vi "fgv_PXI-5110_procon.vi"(7 "cmd":T2, 8 "error in":errorcluster, 11 "data":T1) -> (0 "error out":errorcluster, 3 "queue out":refnum<queue>)   [LabVIEW 2021]
uses:
  ctrl/create-rw-close.ctl
  ctrl/5110_cmd.ctl
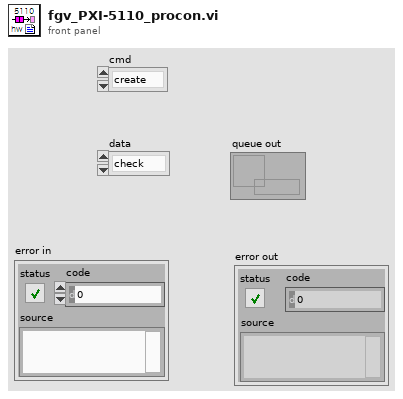
[diagram p1: front panel]
types:
  T1 = typedef "5110_cmd.ctl" = enum16{"check", "run", "stop"}
  T2 = typedef "create-rw-close.ctl" = enum16{"create", "read", "write", "close"}
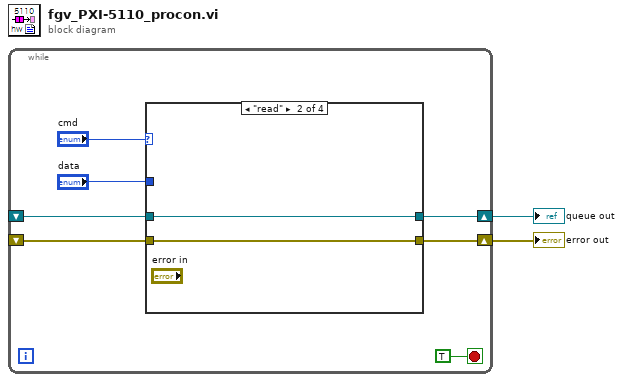
[diagram p0: block diagram]
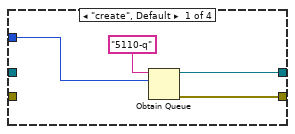
[diagram p2: hidden frame]
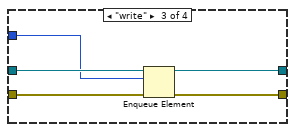
[diagram p3: hidden frame]
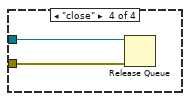
[diagram p4: hidden frame]
diagram:
  n1 = while {
    shift-right: [w7] -> w1
    shift-left: _ -> [w6]
    shift-right: [w5] -> w2
    shift-left: _ -> [w4]
    stop <- TRUE stop-if-true
    n2 = case shown="\"read\"" "cmd" {
      tunnel: [w13 w15 w20 _] -> w7
      tunnel: w6 -> [_ w15 w18 w22]
      tunnel: [w12 w14 w19 _] -> w5
      tunnel: w4 -> [_ w14 w17 w21]
      tunnel: "data" -> [w10 _ w16 _]
      frame "create", Default {
        n3 = Obtain Queue(name (unnamed)="5110-q", element data type=w10) -> (queue out=w13:refnum<queue>, error out=w12:errorcluster)  [unwired: 3 in, 1 out]
      }
      frame "read" {
      }
      frame "write" {
        n4 = Enqueue Element(queue=w18, element=w16, error in (no error)=w17) -> (queue out=w20:refnum<queue>, error out=w19:errorcluster)  [unwired: 1 in, 1 out]
      }
      frame "close" {
        n5 = Release Queue(queue=w22, error in (no error)=w21) -> ()  [unwired: 1 in, 3 out]
      }
    }
  }
  "error out" <- w2
  "queue out" <- w1
